vi "Get 2D Time Stamp.vi"(5 "format string (%s)":string="%s", 7 "key description":string, 8 "sections":string[](array[string]), 9 "time stamp":timestamp[][](array[timestamp]), 11 "info data":string) -> (0 "sections out":string[](array[string]), 1 "found?":bool, 2 "value":timestamp[][](array[timestamp]), 3 "info data out":string)   [LabVIEW 2013, in "infolib.lvlib"]
doc: "Reads matrix of time stamps. If section is entered it searches the key in the section(s)."
uses:
  infolib.lvlib
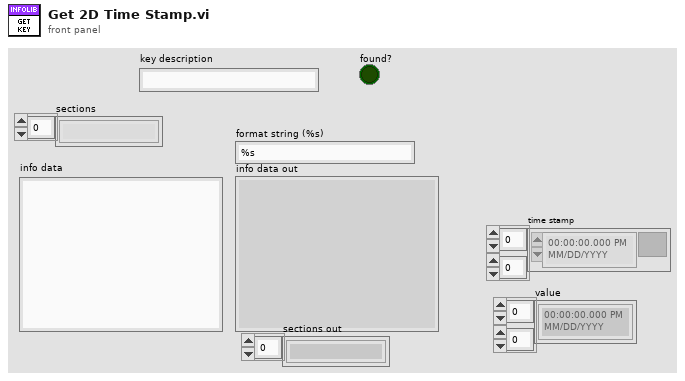
[diagram p1: front panel]
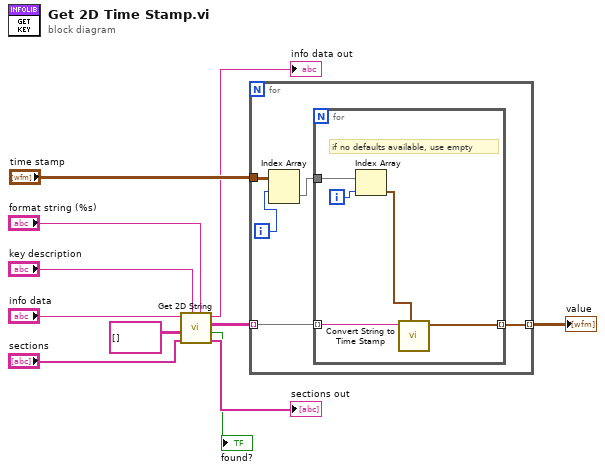
[diagram p0: block diagram]
diagram:
  n1 = call "Get 2D String.vi"("format string (%s)"="format string (%s)", "key description"="key description", "sections"="sections", "string"=string[][] [] ("1D string array"), "info data"="info data") -> ("sections out"=→"sections out":string[], "found?"=→"found?":bool, "value"=w2:string[][], "info data out"=→"info data out":string)  [unwired: 3 in]
  n2 = for {
    tunnel: [w16] -> w11 mode=indexing
    tunnel: "time stamp" -> [w14]
    tunnel: w2 -> [w15] mode=indexing
    i -> [w13]
    n3 = Index Array(array=w14, index (row)=w13) -> (element=w12:timestamp[])  [unwired: 1 in]
    n4 = for {
      tunnel: w12 -> [w21]
      tunnel: w15 -> [w20] mode=indexing
      tunnel: [w18] -> w16 mode=indexing
      i -> [w17]
      # "if no defaults available, use empty"
      n5 = Index Array(array=w21, index=w17) -> (element=w19:timestamp)
      n6 = call "Convert String to Time Stamp.vi"("default value of time stamp"=w19, "string"=w20) -> ("time stamp out"=w18:timestamp)  [unwired: 9 in]
    }
  }
  "value" <- w11
